vi "nanocal -- nuclear schottky fit -- 2x2 -- V9.vi"() -> ()   [LabVIEW 2021] (continued)
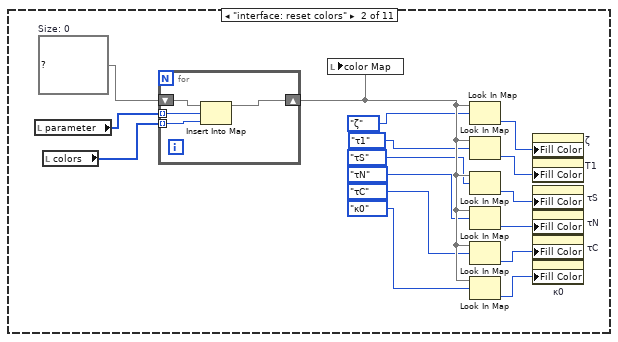
[diagram p3: hidden frame]
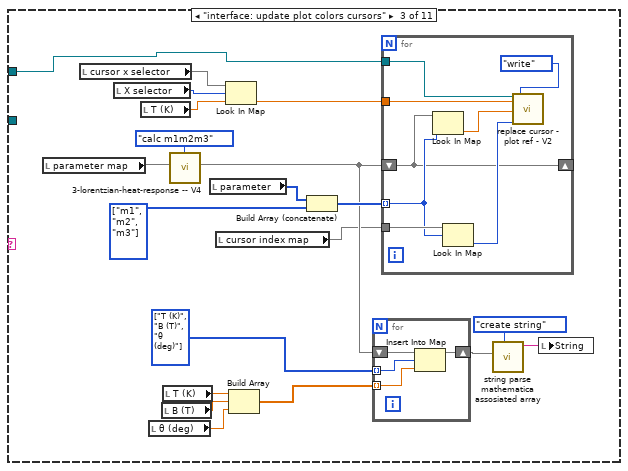
[diagram p4: hidden frame]
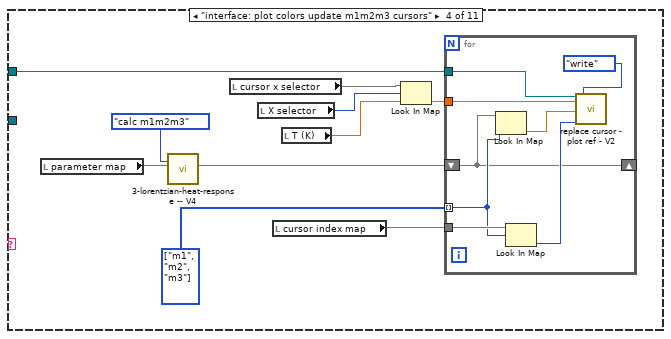
[diagram p5: hidden frame]
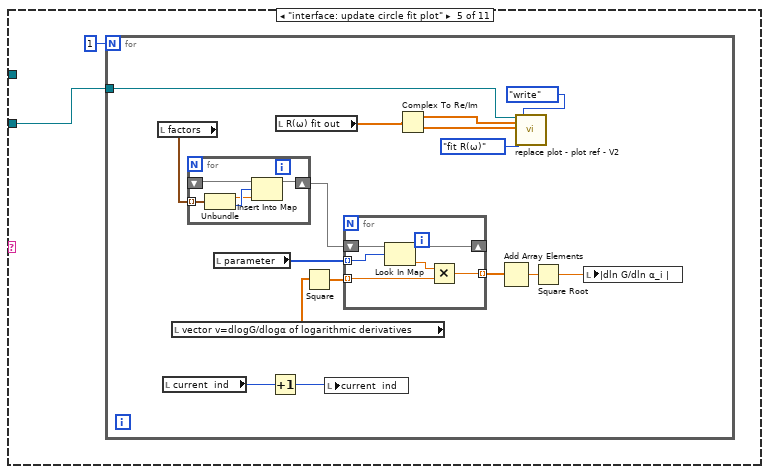
[diagram p6: hidden frame]
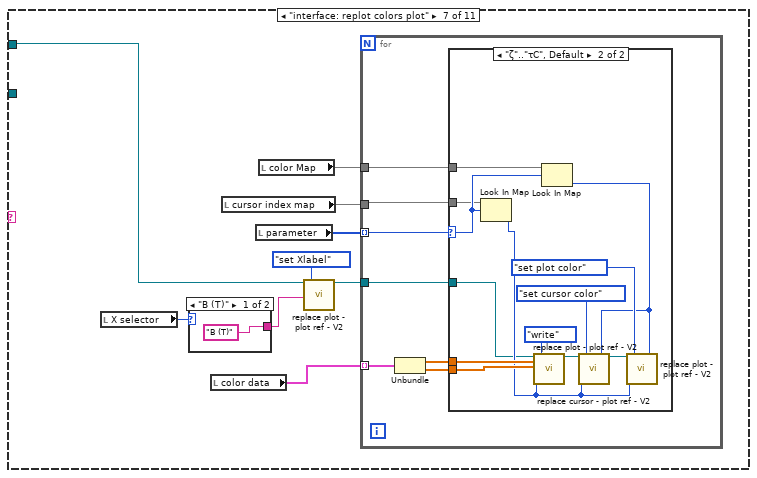
[diagram p8: hidden frame]
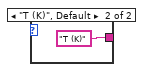
[diagram p9: hidden frame]
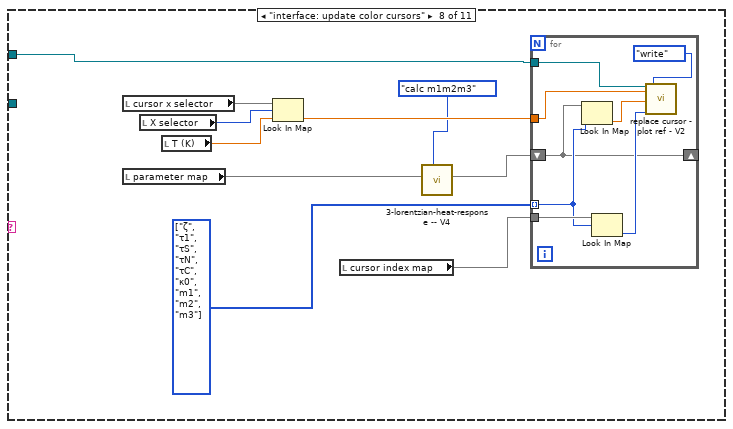
[diagram p11: hidden frame]
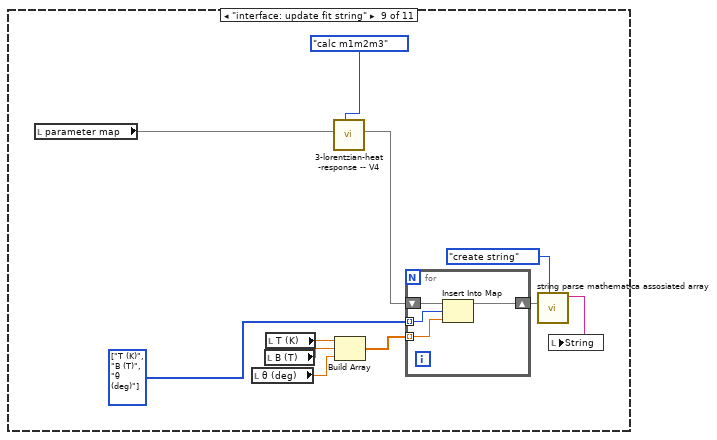
[diagram p12: hidden frame]
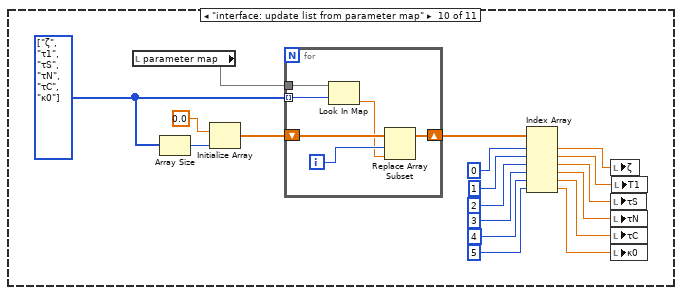
[diagram p13: hidden frame]
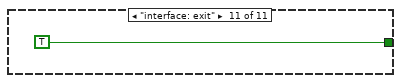
[diagram p14: hidden frame]
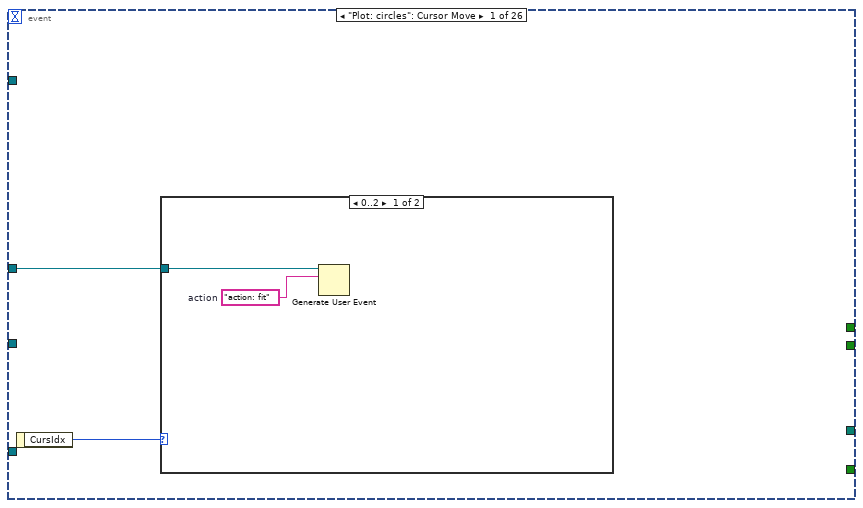
[diagram p15: hidden frame]
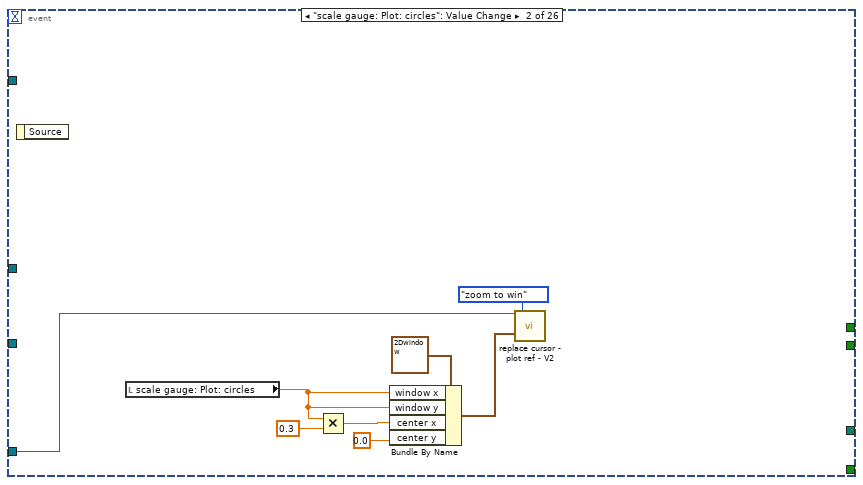
[diagram p17: hidden frame]
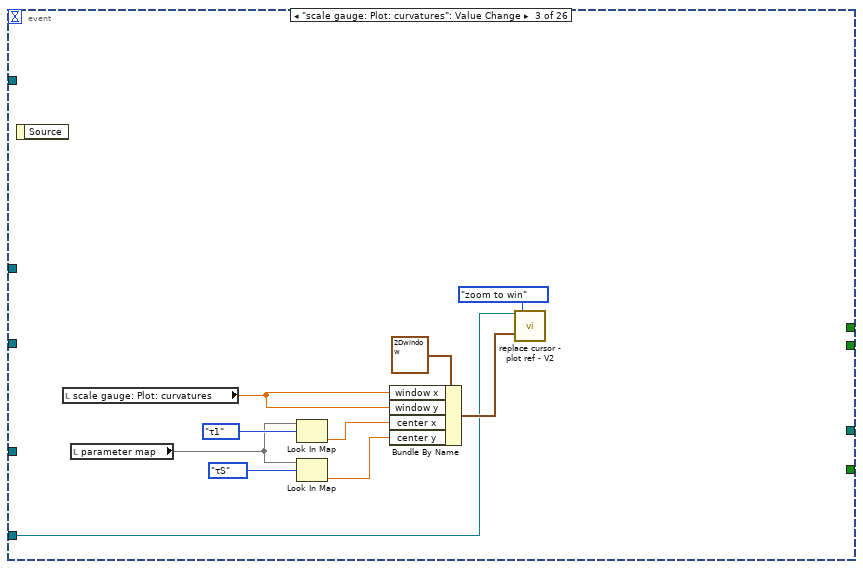
[diagram p18: hidden frame]
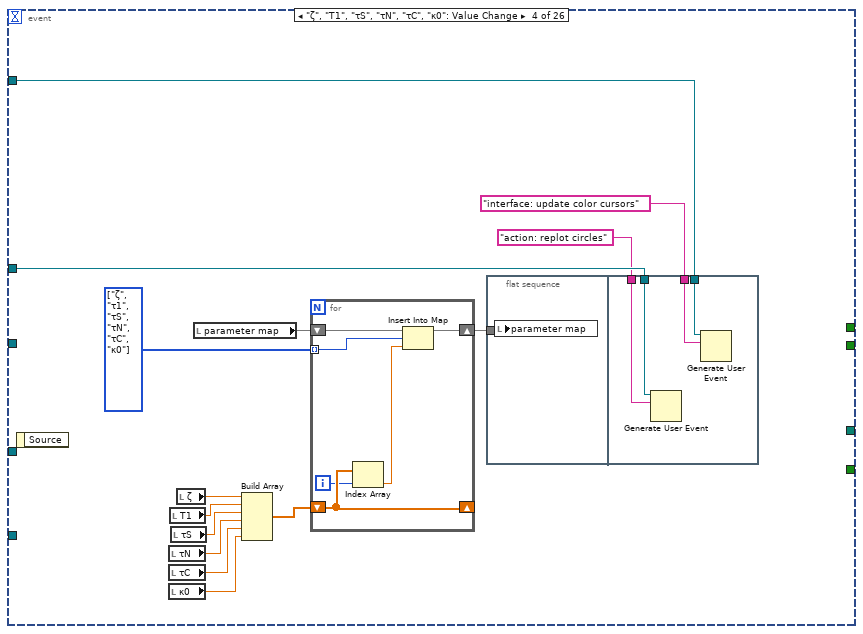
[diagram p19: hidden frame]
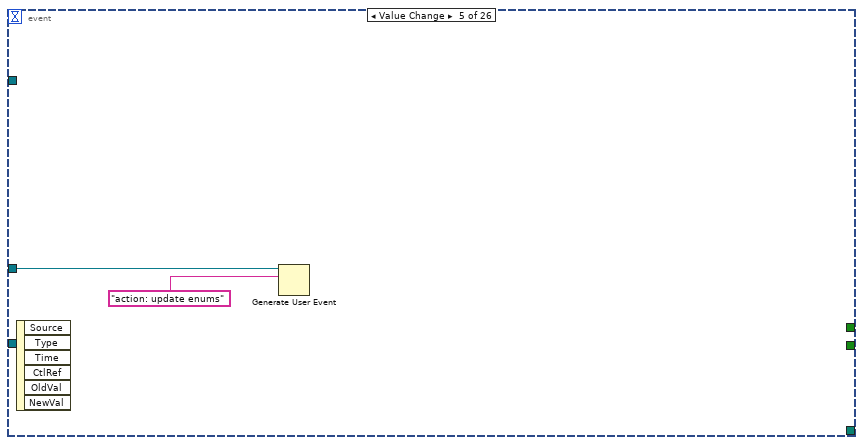
[diagram p20: hidden frame]
            n551 = call "3-lorentzian-heat-response -- V4.vi"("action"=3-lorentzian-heat-response_action."calc m1m2m3", "Map IN"=w1167) -> ("Map OUT"=w1166:map{T2, dbl})  [unwired: 7 in, 2 out]
            n552 = local read "cursor x selector"() -> (w1161:map{T2, dbl})
            n553 = local read "X selector"() -> (w1162:T2)
            n554 = local read "cursor index map"() -> (w1165:map{T2, i32})
            n555 = local read "T (K)"() -> (w1163:dbl)
            n556 = Look In Map(map=w1161, key=w1162, default value=w1163) -> (value=w1164:dbl)  [unwired: 1 out]
            n557 = for {
              tunnel: w1164 -> [w1175]
              tunnel: w1159 -> [w1171] mode=indexing
              tunnel: w1165 -> [w1173]
              shift-right: [w1170] -> _
              shift-left: w1166 -> [w1170]
              tunnel: w1158 -> [w1168]
              n558 = Look In Map(map=w1170, key=w1171) -> (value=w1169:dbl)  [unwired: 1 in, 1 out]
              n559 = Look In Map(map=w1173, key=w1171) -> (value=w1172:i32)  [unwired: 1 in, 1 out]
              n560 = call "replace cursor - plot ref - V2.vi"("Plot ref in"=w1168, "new X"=w1175, "new  Y"=w1169, "cursor index"=w1172, "cursor action"=cursor_action."write") -> ()  [unwired: 11 in, 4 out]
            }
          }
          frame "interface: update circle fit plot" {
            n561 = for {
              N: 1 -> [_]
              tunnel: w1176 -> [w1178]
              n562 = local read "factors"() -> (w1188:cluster{"scaling":dbl, "what":T2}[])
              n563 = local read "current  ind"() -> (w1180:i32)
              n564 = local read "vector v=dlogG/dlogα of logarithmic derivatives"() -> (w1183:dbl[])
              n565 = for {
                shift-right: [w1202] -> w1182
                shift-left: _ -> [w1203]
                tunnel: w1188 -> [w1201] mode=indexing
                n566 = Unbundle(w1201) -> ("scaling"=w1199:dbl, "what"=w1200:T2)
                n567 = Insert Into Map(map in=w1203, key=w1200, value=w1199) -> (map out=w1202:map{T2, dbl})  [unwired: 2 out]
              }
              n568 = local read "parameter"() -> (w1184:T2[])
              n569 = Increment(x=w1180) -> (x+1=w1179:i32)
              n570 = local read "R(ω) fit out"() -> (w1193:cdb[])
              n571 = Square(x=w1183) -> (x^2=w1186:dbl[])
              n572 = local write "current  ind"(w1179) -> ()
              n573 = for {
                tunnel: w1184 -> [w1198] mode=indexing
                shift-right: [w1197] -> _
                shift-left: w1182 -> [w1197]
                tunnel: w1186 -> [w1195] mode=indexing
                tunnel: [w1194] -> w1185 mode=indexing
                n574 = Look In Map(map=w1197, key=w1198) -> (value=w1196:dbl)  [unwired: 1 in, 1 out]
                n575 = Multiply(x=w1196, y=w1195) -> (x*y=w1194:dbl)
              }
              n576 = Complex To Re/Im(x + iy=w1193) -> (x=w1191:dbl[], y=w1192:dbl[])
              n577 = Add Array Elements(numeric array=w1185) -> (sum=w1187:dbl)
              n578 = call "replace plot - plot ref - V2.vi"("Plot ref in"=w1178, "Array X IN"=w1191, "Array Y IN"=w1192, "plot index"=enum16{"data R(ω)", "fit R(ω)"}."fit R(ω)" ("Plost: sweep window"), "cursor action"=cursor_action."write") -> ()  [unwired: 11 in, 4 out]
              n579 = Square Root(x=w1187) -> (sqrt(x)=w1181:dbl)
              n580 = local write "|dln G/dln α_i |"(w1181) -> ()
            }
          }
          frame "interface: update curvature plot" {
            n581 = local read "error goodness weighting"() -> (w1205:T5)
            n582 = local read "newton parameters"() -> (w1206:T3)
            n583 = Bundle By Name(cluster=w1206, "weighting"=w1205) -> (w1204:T3)
            n584 = control-ref of="Plot: curvature"() -> (w1208:refnum<vi>)
            n585 = case shown="True" "update  as you fit" {
              tunnel: w1208 -> [_ _]
              tunnel: w1204 -> [_ w1213]
              frame False {
              }
              frame True {
                n586 = local read "curvature triplets"() -> (w1216:T11[])
                n587 = local read "parameter map"() -> (w1218:map{T2, dbl})
                n588 = local read "sampling size(%)"() -> (w1214:dbl)
                n589 = local read "error-mode"() -> (w1209:T15)
                n590 = call "nanocal -- publish -- freq scan V2.vi"("publisher action"=publisher_action."get") -> ("data"=w1215:T34)  [unwired: 7 in, 3 out]
                n591 = call "nanocal -- generate 3D curvature ellipsoid --  V4.vi"("sampling vicinity size (%)"=w1214, "error mode"=w1209, "newton parameters"=w1213, "data"=w1215, "Curvature triplet array IN"=w1216, "parameter map"=w1218) -> ("Curvature triplet array OUT"=w1212:T11[])  [unwired: 5 in]
                n592 = Index Array(array=w1212, index=0) -> (element=w1210:T11)
                n593 = Unbundle By Name(w1210) -> ()  [unwired: 1 out]
                n594 = local write "curvature triplets"(w1212) -> ()
              }
            }
          }
          frame "interface: replot colors plot" {
            n595 = local read "X selector"() -> (w1220:T2)
            n596 = case shown="\"B (T)\"" w1220 {
              tunnel: ["B (T)" "T (K)"] -> w1226
              frame "B (T)" {
              }
              frame "T (K)", Default {
              }
            }
            n597 = local read "color data"() -> (w1223:cluster{"Array":dbl[], "Array":dbl[]}[])
            n598 = local read "cursor index map"() -> (w1221:map{T2, i32})
            n599 = local read "parameter"() -> (w1227:T2[])
            n600 = local read "color Map"() -> (w1222:map{T2, u32})
            n601 = call "replace plot - plot ref - V2.vi"("Plot ref in"=w1219, "text"=w1226, "cursor action"=cursor_action."set Xlabel") -> ("Plot ref out"=w1224:refnum<vi>)  [unwired: 13 in, 3 out]
            n602 = for {
              tunnel: w1227 -> [w1236] mode=indexing
              tunnel: w1224 -> [w1235]
              tunnel: w1223 -> [w1234] mode=indexing
              tunnel: w1222 -> [w1231]
              tunnel: w1221 -> [w1230]
              n603 = Unbundle(w1234) -> ("Array"=w1232:dbl[], "Array"=w1233:dbl[])
              n604 = case shown="\"ζ\"..\"τC\", Default" w1236 {
                selector: w1236 -> [_ w1245]
                tunnel: w1232 -> [_ w1247]
                tunnel: w1233 -> [_ w1246]
                tunnel: w1231 -> [_ w1244]
                tunnel: w1230 -> [_ w1243]
                tunnel: w1235 -> [_ w1237]
                frame "κ0" {
                }
                frame "ζ".."τC", Default {
                  n605 = Look In Map(map=w1243, key=w1245) -> (value=w1239:i32)  [unwired: 1 in, 1 out]
                  n606 = call "replace plot - plot ref - V2.vi"("Plot ref in"=w1237, "Array X IN"=w1247, "Array Y IN"=w1246, "plot index"=w1239, "cursor action"=cursor_action."write") -> ("Plot ref out"=w1242:refnum<vi>)  [unwired: 11 in, 3 out]
                  n607 = Look In Map(map=w1244, key=w1245) -> (value=w1238:u32)  [unwired: 1 in, 1 out]
                  n608 = call "replace cursor - plot ref - V2.vi"("Plot ref in"=w1242, "cursor index"=w1239, "cursor action"=cursor_action."set cursor color", "Color Box"=w1238) -> ("Plot ref out"=w1241:refnum<vi>)  [unwired: 12 in, 3 out]
                  n609 = call "replace plot - plot ref - V2.vi"("Plot ref in"=w1241, "plot index"=w1239, "cursor action"=cursor_action."set plot color", "Color Box"=w1238) -> ()  [unwired: 12 in, 4 out]
                }
              }
            }
          }
          frame "interface: update color cursors" {
            w1252 = T2[] [enum."ζ", enum."τ1", enum."τS", enum."τN", enum."τC", enum."κ0", enum."m1", enum."m2", enum."m3"] items=["ζ", "τ1", "τS", "τN", "τC", "κ0", "m1", "m2", "m3", "T (K)", "B (T)", "θ (deg)", "side (S|R)", "set of (B|T)", "Re(offset)", "Im(offset)", "στ1", "στ1-", "στ1+", "στS", "στS-", "στS+", "στN", "στN-", "στN+", "τ11", "τ12", "τ21", "τ22", "τN1", "τN2"]
            n610 = local read "cursor x selector"() -> (w1254:map{T2, dbl})
            n611 = local read "parameter map"() -> (w1251:map{T2, dbl})
            n612 = local read "X selector"() -> (w1255:T2)
            n613 = local read "T (K)"() -> (w1256:dbl)
            n614 = Look In Map(map=w1254, key=w1255, default value=w1256) -> (value=w1257:dbl)  [unwired: 1 out]
            n615 = local read "cursor index map"() -> (w1258:map{T2, i32})
            n616 = call "3-lorentzian-heat-response -- V4.vi"("action"=3-lorentzian-heat-response_action."calc m1m2m3", "Map IN"=w1251) -> ("Map OUT"=w1259:map{T2, dbl})  [unwired: 7 in, 2 out]
            n617 = for {
              tunnel: w1257 -> [w1267]
              tunnel: w1250 -> [w1266]
              tunnel: w1252 -> [w1262] mode=indexing
              tunnel: w1258 -> [w1264]
              shift-right: [w1261] -> _
              shift-left: w1259 -> [w1261]
              n618 = Look In Map(map=w1261, key=w1262) -> (value=w1260:dbl)  [unwired: 1 in, 1 out]
              n619 = Look In Map(map=w1264, key=w1262) -> (value=w1263:i32)  [unwired: 1 in, 1 out]
              n620 = call "replace cursor - plot ref - V2.vi"("Plot ref in"=w1266, "new X"=w1267, "new  Y"=w1260, "cursor index"=w1263, "cursor action"=cursor_action."write") -> ()  [unwired: 11 in, 4 out]
            }
          }
          frame "interface: update fit string" {
            w1270 = T2[] [enum."T (K)", enum."B (T)", enum."θ (deg)"] items=["ζ", "τ1", "τS", "τN", "τC", "κ0", "m1", "m2", "m3", "T (K)", "B (T)", "θ (deg)", "side (S|R)", "set of (B|T)", "Re(offset)", "Im(offset)", "στ1", "στ1-", "στ1+", "στS", "στS-", "στS+", "στN", "στN-", "στN+", "τ11", "τ12", "τ21", "τ22", "τN1", "τN2"]
            n621 = local read "parameter map"() -> (w1268:map{T2, dbl})
            n622 = local read "θ (deg)"() -> (w1274:dbl)
            n623 = local read "B (T)"() -> (w1273:dbl)
            n624 = local read "T (K)"() -> (w1272:dbl)
            n625 = call "3-lorentzian-heat-response -- V4.vi"("action"=3-lorentzian-heat-response_action."calc m1m2m3", "Map IN"=w1268) -> ("Map OUT"=w1275:map{T2, dbl})  [unwired: 7 in, 2 out]
            n626 = Build Array(w1272, w1273, w1274) -> (w1276:dbl[])
            n627 = for {
              shift-right: [w1281] -> w1277
              shift-left: w1275 -> [w1282]
              tunnel: w1270 -> [w1280] mode=indexing
              tunnel: w1276 -> [w1279] mode=indexing
              n628 = Insert Into Map(map in=w1282, key=w1280, value=w1279) -> (map out=w1281:map{T2, dbl})  [unwired: 2 out]
            }
            n629 = call "string parse mathematica assosiated array.vi"("action"=mathematica_string_map_action."create string" ("derivative"), "map IN"=w1277) -> ("String OUT"=w1278:string)  [unwired: 8 in, 1 out]
            n630 = local write "String"(w1278) -> ()
          }
          frame "interface: update list from parameter map" {
            w1284 = T2[] [enum."ζ", enum."τ1", enum."τS", enum."τN", enum."τC", enum."κ0"] items=["ζ", "τ1", "τS", "τN", "τC", "κ0", "m1", "m2", "m3", "T (K)", "B (T)", "θ (deg)", "side (S|R)", "set of (B|T)", "Re(offset)", "Im(offset)", "στ1", "στ1-", "στ1+", "στS", "στS-", "στS+", "στN", "στN-", "στN+", "τ11", "τ12", "τ21", "τ22", "τN1", "τN2"]
            n631 = local read "parameter map"() -> (w1287:map{T2, dbl})
            n632 = Array Size(array=w1284) -> (size(s)=w1283:i32)
            n633 = Initialize Array(0.0 ("new X"), w1283) -> (w1286:dbl[])
            n634 = for {
              tunnel: w1284 -> [w1305] mode=indexing
              tunnel: w1287 -> [w1306]
              shift-right: [w1303] -> w1289
              shift-left: w1286 -> [w1304]
              i -> [w1302]
              n635 = Look In Map(map=w1306, key=w1305) -> (value=w1301:dbl)  [unwired: 1 in, 1 out]
              n636 = Replace Array Subset(array=w1304, new element=w1301, index=w1302) -> (w1303:dbl[])
            }
            n637 = Index Array(array=w1289, index #1=0 ("index"), index #2=1 ("index"), index #3=2 ("index"), index #4=3 ("index"), index #5=4 ("index"), index #6=5 ("index")) -> (element #1=w1288:dbl, element #2=w1296:dbl, element #3=w1297:dbl, element #4=w1298:dbl, element #5=w1299:dbl, element #6=w1300:dbl)
            n638 = local write "ζ"(w1288) -> ()
            n639 = local write "τS"(w1297) -> ()
            n640 = local write "τN"(w1298) -> ()
            n641 = local write "τC"(w1299) -> ()
            n642 = local write "κ0"(w1300) -> ()
            n643 = local write "T1"(w1296) -> ()
          }
          frame "interface: exit" {
          }
        }
      }
    }
  }
  n644 = while "interface events" {
    tunnel: w9 -> [w1313]
    tunnel: w38 -> [w1312]
    tunnel: w35 -> [w1311]
    tunnel: w10 -> [w1310]
    tunnel: w3 -> [w1308]
    stop <- FALSE stop-if-true
    n645 = event shown="[11] \"offset Re offset Im\", \"|ω| < limit (Hz)\", \"cspan\": Value Change" {
      selector: _ -> [_ _ _ _ _ _ _ _ _ _ _ _ _ _ _ _ _ _ _ _ _ _ _ _ _ _]
      dyn-events: _ -> [_ _ _ _ _ _ _ _ _ _ _ _ _ _ _ _ _ _ _ _ _ _ _ _ _ _]
      timeout: _ -> [_ _ _ _ _ _ _ _ _ _ _ _ _ _ _ _ _ _ _ _ _ _ _ _ _ _]
      tunnel: w1313 -> [w1314 _ _ w1337 w1361 _ w1386 w1392 _ w1396 w1398 w1400 w1403 w1410 w1506 w1527 w1547 w1549 w1553 w1556 w1559 w1562 w1570 w1574 w1576 w1579]
      tunnel: [_ _ _ _ _ _ _ _ _ "load! :l" _ _ _ _ _ _ _ _ _ _ _ _ _ _ _ _] -> _
      tunnel: [_ _ _ _ _ _ "go / pause!" _ _ _ _ _ "parse! :p" _ _ _ "Math→τ! :q" _ "τ→Math! :p" "Math→ string OUT! :s" "generate empty string from filelist !" "string IN → Math!" _ _ "plot landscape!" _] -> _
      tunnel: w1312 -> [_ w1318 _ _ _ w1363 _ _ _ _ _ _ _ w1406 _ _ _ _ _ _ _ _ _ _ _ _]
      tunnel: w1311 -> [_ _ _ _ _ _ _ _ _ _ _ _ _ _ w1514 w1535 _ _ _ _ _ _ _ _ _ _]
      tunnel: [_ _ _ _ _ _ _ _ _ _ "Read from file" _ _ _ _ _ _ _ _ _ _ _ _ _ _ _] -> _
      tunnel: [_ _ _ _ _ _ _ _ _ _ _ _ _ _ _ _ _ "load default values" _ _ _ _ _ _ _ _] -> _
      tunnel: w1310 -> [_ _ _ w1339 _ _ _ _ _ _ _ _ _ _ w1504 w1525 _ _ _ _ _ _ _ _ _ _]
      tunnel: w1308 -> [_ _ w1332 _ _ _ _ _ _ _ _ _ _ w1405 _ _ _ _ _ _ _ _ _ _ _ _]
      event "Plot: circles": Cursor Move {
        n646 = event-data() -> ("CursIdx"=w1315:i32)  [unwired: 1 in]
        n647 = case shown="0..2" w1315 {
          tunnel: w1314 -> [w1317 _]
          frame 0..2 {
            w1316 = "action: fit"  # action
            n648 = Generate User Event(user event=w1317, event data cluster=w1316) -> ()  [unwired: 2 in, 2 out]
          }
          frame 3..5, Default {
          }
        }
      }
      event "scale gauge: Plot: circles": Value Change {
        n649 = event-data() -> ()  [unwired: 1 in, 1 out]
        n650 = local read "scale gauge: Plot: circles"() -> (w1324:dbl)
        n651 = Multiply(x=w1324, y=0.3) -> (x*y=w1325:dbl)
        n652 = Bundle By Name(cluster=T37 {"window y"=0.0021014740628288917, "center x"=44850.89441339177, "center y"=2.5658109925320947, "window x"=17480.201988350764} ("window IN"), "window x"=w1324, "window y"=w1324, "center x"=w1325, "center y"=0.0) -> (w1323:T37)
        n653 = call "replace cursor - plot ref - V2.vi"("Plot ref in"=w1318, "window IN"=w1323, "cursor action"=cursor_action."zoom to win") -> ()  [unwired: 13 in, 4 out]
      }
      event "scale gauge: Plot: curvatures": Value Change {
        n654 = event-data() -> ()  [unwired: 1 in, 1 out]
        n655 = local read "scale gauge: Plot: curvatures"() -> (w1328:dbl)
        n656 = local read "parameter map"() -> (w1329:map{T2, dbl})
        n657 = Look In Map(map=w1329, key=3-lorentzian-parameters."τ1") -> (value=w1327:dbl)  [unwired: 1 in, 1 out]
        n658 = Look In Map(map=w1329, key=3-lorentzian-parameters."τS") -> (value=w1326:dbl)  [unwired: 1 in, 1 out]
        n659 = Bundle By Name(cluster=T37 {"window y"=0.0021014740628288917, "center x"=44850.89441339177, "center y"=2.5658109925320947, "window x"=17480.201988350764} ("window IN"), "window x"=w1328, "window y"=w1328, "center x"=w1327, "center y"=w1326) -> (w1335:T37)
        n660 = call "replace cursor - plot ref - V2.vi"("Plot ref in"=w1332, "window IN"=w1335, "cursor action"=cursor_action."zoom to win") -> ()  [unwired: 13 in, 4 out]
      }
      event "ζ", "T1", "τS", "τN", "τC", "κ0": Value Change {
        w1340 = T2[] [enum."ζ", enum."τ1", enum."τS", enum."τN", enum."τC", enum."κ0"] items=["ζ", "τ1", "τS", "τN", "τC", "κ0", "m1", "m2", "m3", "T (K)", "B (T)", "θ (deg)", "side (S|R)", "set of (B|T)", "Re(offset)", "Im(offset)", "στ1", "στ1-", "στ1+", "στS", "στS-", "στS+", "στN", "στN-", "στN+", "τ11", "τ12", "τ21", "τ22", "τN1", "τN2"]
        n661 = event-data() -> ()  [unwired: 1 in, 1 out]
        n662 = local read "τN"() -> (w1346:dbl)
        n663 = local read "τC"() -> (w1345:dbl)
        n664 = local read "κ0"() -> (w1344:dbl)
        n665 = local read "T1"() -> (w1348:dbl)
        n666 = local read "τS"() -> (w1347:dbl)
        n667 = local read "ζ"() -> (w1349:dbl)
        n668 = local read "parameter map"() -> (w1341:map{T2, dbl})
        n669 = Build Array(w1349, w1348, w1347, w1346, w1345, w1344) -> (w1343:dbl[])
        n670 = for {
          tunnel: w1340 -> [w1355] mode=indexing
          shift-right: [w1360] -> _
          shift-left: w1343 -> [w1360]
          shift-right: [w1357] -> w1342
          shift-left: w1341 -> [w1358]
          i -> [w1359]
          n671 = Index Array(array=w1360, index=w1359) -> (element=w1356:dbl)
          n672 = Insert Into Map(map in=w1358, key=w1355, value=w1356) -> (map out=w1357:map{T2, dbl})  [unwired: 2 out]
        }
        n673 = flat-sequence {
          tunnel: w1342 -> [w1350]
          tunnel: w1339 -> [w1354]
          tunnel: "interface: update color cursors" ("event data") -> [w1353]
          tunnel: w1337 -> [w1352]
          tunnel: "action: replot circles" ("event data") -> [w1351]
          frame #0 {
            n674 = local write "parameter map"(w1350) -> ()
          }
          frame #1 {
            n675 = Generate User Event(user event=w1352, event data cluster=w1351) -> ()  [unwired: 2 in, 2 out]
            n676 = Generate User Event(user event=w1354, event data cluster=w1353) -> ()  [unwired: 2 in, 2 out]
          }
        }
      }
      event Value Change {
        n677 = event-data() -> ()  [unwired: 1 in, 6 out]
        n678 = Generate User Event(user event=w1361, event data cluster="action: update enums" ("event data")) -> ()  [unwired: 2 in, 2 out]
      }
      event "ω0 (rad/sec)": Value Change {
        n679 = event-data() -> ()  [unwired: 1 in, 1 out]
        n680 = local read "parameter map"() -> (w1365:map{T2, dbl})
        n681 = call "nanocal -- publish -- freq scan V2.vi"("publisher action"=publisher_action."get") -> ("z out (V)"=w1383:cdb[], "ω out (Hz)"=w1378:dbl[])  [unwired: 7 in, 2 out]
        n682 = Divide(x="ω0 (rad/sec)", y=6.283185307179586) -> (x/y=w1376:dbl)
        n683 = call "3-lorentzian-heat-response -- V4.vi"("action"=3-lorentzian-heat-response_action."calc R", "Map IN"=w1365, "omega IN (rad/sec)"="ω0 (rad/sec)") -> ("Romega"=w1375:cdb)  [unwired: 6 in, 2 out]
        n684 = Threshold 1D Array(2:w1376, 3:w1378) -> (0:w1377:dbl)  [unwired: 1 in]
        n685 = Complex To Re/Im(x + iy=w1375) -> (x=w1373:dbl, y=w1374:dbl)
        n686 = Index Array(array=w1383, index=w1377) -> (element=w1380:cdb)
        n687 = call "replace cursor - plot ref - V2.vi"("Plot ref in"=w1363, "new X"=w1373, "new  Y"=w1374, "cursor index"=0, "cursor action"=cursor_action."write") -> ("Plot ref out"=w1379:refnum<vi>)  [unwired: 11 in, 3 out]
        n688 = Complex To Re/Im(x + iy=w1380) -> (x=w1381:dbl, y=w1382:dbl)
        n689 = call "replace cursor - plot ref - V2.vi"("Plot ref in"=w1379, "new X"=w1381, "new  Y"=w1382, "cursor index"=1, "cursor action"=cursor_action."write") -> ()  [unwired: 11 in, 4 out]
      }
      event "go / pause!": Value Change {
        n690 = event-data() -> ()  [unwired: 1 in, 1 out]
        n691 = local read "newton is active"() -> (w1384:bool)
        n692 = case shown="True" w1384 {
          tunnel: w1386 -> [_ w1391]
          tunnel: [FALSE TRUE] -> w1385
          frame True {
          }
          frame False {
            n693 = Generate User Event(user event=w1391, event data cluster="action: gradient step" ("event data")) -> ()  [unwired: 2 in, 2 out]
          }
        }
        n694 = local write "newton is active"(w1385) -> ()
      }
      event "selector": Value Change {
        n695 = event-data() -> ()  [unwired: 1 in, 1 out]
        n696 = Generate User Event(user event=w1392, event data cluster="action: update state of selectors" ("event data")) -> ()  [unwired: 2 in, 2 out]
      }
      event "Plot: circles": Cursor Release {
        n697 = event-data() -> ()  [unwired: 1 in, 1 out]
      }
      event "load! :l": Value Change {
        n698 = event-data() -> ()  [unwired: 1 in, 6 out]
        n699 = Generate User Event "action User Event"(user event=w1396, event data cluster="action: read from file" ("event data")) -> ()  [unwired: 2 in, 2 out]
      }
      event "Read from file": Value Change {
        n700 = event-data() -> ()  [unwired: 1 in, 6 out]
        n701 = Generate User Event ("action User Event")(user event=w1398, event data cluster="action: read from file" ("event data")) -> ()  [unwired: 2 in, 2 out]
      }
      event "offset Re\noffset Im", "|ω| < limit (Hz)", "cspan": Value Change {
        n702 = event-data() -> ()  [unwired: 1 in, 6 out]
        n703 = Generate User Event "action User Event"(user event=w1400, event data cluster="action: read from file" ("event data")) -> ()  [unwired: 2 in, 2 out]
      }
      event "parse! :p": Value Change {
        n704 = event-data() -> ()  [unwired: 1 in, 6 out]
        n705 = Generate User Event "action User Event"(user event=w1403, event data cluster="action: parse string" ("event data")) -> ()  [unwired: 2 in, 2 out]
      }
      event Key Down {
        n706 = event-data() -> ("Char"=w1408:i16, "VKey"=w1411:T38)  [unwired: 1 in]
        n707 = Build Array(w1408) -> (w1409:i16[])
        n708 = Byte Array To String(unsigned byte array=w1409) -> (string=w1407:string)
        n709 = case shown="\"ASCII\", Default" w1411 {
          selector: w1411 -> [_ _ _ _ _ w1498]
          tunnel: w1410 -> [w1415 _ w1491 _ _ _]
          tunnel: w1407 -> [w1414 _ _ _ _ _]
          tunnel: w1406 -> [w1413 _ _ _ _ w1497]
          tunnel: w1405 -> [w1412 _ _ _ _ w1496]
          frame "ASCII", Default {
            n710 = case shown="\"b\"" w1414 {
              selector: w1414 -> [_ _ _ _ _ _ w1440 w1450 _ _ _ _ w1470 _]
              tunnel: w1415 -> [_ _ w1416 w1418 w1422 _ _ _ _ w1461 w1464 w1466 w1468 w1489]
              tunnel: w1413 -> [_ _ _ _ _ w1436 _ _ _ _ _ _ _ _]
              tunnel: w1412 -> [_ _ _ _ _ w1429 _ _ _ _ _ _ _ _]
              frame "0", Default {
              }
              frame "a" {
              }
              frame "s" {
                n711 = Generate User Event(user event=w1416, event data cluster="action: write mathematica string" ("event data")) -> ()  [unwired: 2 in, 2 out]
              }
              frame "l" {
                n712 = Generate User Event(user event=w1418, event data cluster="action: read from file" ("event data")) -> ()  [unwired: 2 in, 2 out]
              }
              frame " " {
                n713 = local read "newton is active"() -> (w1421:bool)
                n714 = case shown="False" w1421 {
                  selector: w1421 -> [w1424 w1426]
                  tunnel: w1422 -> [_ w1428]
                  tunnel: [w1423 w1425] -> w1420
                  frame True {
                    n715 = Not(x=w1424) -> (.not. x?=w1423:bool)
                  }
                  frame False {
                    n716 = Generate User Event(user event=w1428, event data cluster="action: gradient step" ("event data")) -> ()  [unwired: 2 in, 2 out]
                    n717 = Not(x=w1426) -> (.not. x?=w1425:bool)
                  }
                }
                n718 = local write "newton is active"(w1420) -> ()
              }
              frame "?" {
                # "?"
                n719 = call "replace cursor - plot ref - V2.vi"("Plot ref in"=w1436, "cursor action"=cursor_action."zoom to win") -> ("Plot ref out"=w1435:refnum<vi>)  [unwired: 14 in, 3 out]
                n720 = call "replace cursor - plot ref - V2.vi"("Plot ref in"=w1435, "cursor action"=cursor_action."smart zoom out&aspect") -> ()  [unwired: 14 in, 4 out]
                n721 = call "replace cursor - plot ref - V2.vi"("Plot ref in"=w1429, "cursor action"=cursor_action."zoom to win") -> ("Plot ref out"=w1432:refnum<vi>)  [unwired: 14 in, 3 out]
                n722 = call "replace cursor - plot ref - V2.vi"("Plot ref in"=w1432, "cursor action"=cursor_action."smart zoom out&aspect") -> ()  [unwired: 14 in, 4 out]
              }
              frame ",", "." {
                n723 = local read "newton parameters"() -> (w1438:T3)
                n724 = case shown="\".\"" w1440 {
                  tunnel: [0.7 1.0 1.5] -> w1439
                  frame "," {
                  }
                  frame "0", Default {
                  }
                  frame "." {
                  }
                }
                n725 = in-place {
                  in-place-border: w1439 -> [w1443]
                  n726 = in-place-cluster #7(w1438) -> ("PID-P"=w1441:dbl)
                  n727 = Multiply(x=w1443, y=w1441) -> (x*y=w1442:dbl)
                  n728 = in-place-cluster #7("PID-P"=w1442) -> (w1437:T3)
                }
                n729 = local write "newton parameters"(w1437) -> ()
              }
              frame "<", ">" {
                n730 = local read "newton parameters"() -> (w1448:T3)
                n731 = case shown="\"<\"" w1450 {
                  tunnel: [-5 0 5] -> w1449
                  frame "<" {
                  }
                  frame "0", Default {
                  }
                  frame ">" {
                  }
                }
                n732 = in-place {
                  in-place-border: w1449 -> [w1456]
                  n733 = in-place-cluster #8(w1448) -> ("PID-I"=w1455:i32)
                  n734 = Add(x=w1456, y=w1455) -> (x+y=w1454:i32)
                  n735 = In Range and Coerce(upper limit=100, x=w1454, lower limit=2) -> (coerced(x)=w1451:i32)  [unwired: 1 out]
                  n736 = in-place-cluster #8("PID-I"=w1451) -> (w1447:T3)
                }
                n737 = local write "newton parameters"(w1447) -> ()
              }
              frame "b" {
                n738 = local read "String"() -> (w1460:string)
                n739 = local write "backup string :b"(w1460) -> ()
              }
              frame "u" {
                n740 = Generate User Event(user event=w1461, event data cluster="ignoreaction: uco" ("event data")) -> ()  [unwired: 2 in, 2 out]
              }
              frame "p" {
                n741 = Generate User Event ("action User Event")(user event=w1464, event data cluster="action: copy to math" ("event data")) -> ()  [unwired: 2 in, 2 out]
              }
              frame "q" {
                n742 = Generate User Event ("action User Event")(user event=w1466, event data cluster="action: copy from math" ("event data")) -> ()  [unwired: 2 in, 2 out]
              }
              frame "\\", "|" {
                n743 = for {
                  N: 1 -> [_]
                  tunnel: w1470 -> [w1484]
                  tunnel: w1468 -> [w1483]
                  tunnel: [w1483] -> w1467
                  n744 = local read "selection :|\\"() -> (w1476:u16)
                  n745 = property on="selection :|\\" class="Ring (strict)"() -> ("NumItems"=w1474:u32)  [unwired: 2 in, 2 out]
                  n746 = To Long Integer(number=w1476) -> (32bit integer=w1475:i32)
                  n747 = case shown="\"|\", Default" w1484 {
                    tunnel: w1475 -> [w1486 w1488]
                    tunnel: [w1485 w1487] -> w1480
                    frame "|", Default {
                      n748 = Decrement(x=w1486) -> (x-1=w1485:i32)
                    }
                    frame "\\" {
                      n749 = Increment(x=w1488) -> (x+1=w1487:i32)
                    }
                  }
                  n750 = To Long Integer(number=w1474) -> (32bit integer=w1473:i32)
                  n751 = Greater Or Equal?(x=w1480, y=w1473) -> (x >= y?=w1482:bool)
                  n752 = Select(t=u16 0 ("lower limit"), s=w1482, f=w1480) -> (s? t:f=w1477:i32)
                  n753 = Decrement(x=w1473) -> (x-1=w1478:i32)
                  n754 = Less Than 0?(x=w1477) -> (x < 0?=w1479:bool)
                  n755 = Select(t=w1478, s=w1479, f=w1477) -> (s? t:f=w1472:i32)
                  n756 = local write "selection :|\\"(w1472) -> ()
                }
                n757 = Generate User Event ("action User Event")(user event=w1467, event data cluster="action: constrained filenames select" ("event data")) -> ()  [unwired: 2 in, 2 out]
              }
              frame "m" {
                n758 = Generate User Event ("action User Event")(user event=w1489, event data cluster="action: copy from math" ("event data")) -> ()  [unwired: 2 in, 2 out]
              }
            }
          }
          frame "PageUp" {
          }
          frame "Enter" {
            n759 = Generate User Event ("action User Event")(user event=w1491, event data cluster="action: new sweep" ("event data")) -> (user event out=w1492:refnum<user-event>)  [unwired: 2 in, 1 out]
            n760 = Generate User Event ("action User Event")(user event=w1492, event data cluster="action: replot colors" ("event data")) -> ()  [unwired: 2 in, 2 out]
          }
          frame "Caps" {
          }
          frame "PageDown" {
          }
          frame "Up".."Right" {
            n761 = case shown="\"Down\"" w1498 {
              tunnel: [cursor_action."zoom in 20%" ("cursor action") cursor_action."zoom out 20%" ("cursor action") cursor_action."zoom out 20%" ("cursor action") cursor_action."zoom in 20%" ("cursor action")] -> w1495
              frame "Up", Default {
              }
              frame "Down" {
              }
              frame "Left" {
              }
              frame "Right" {
              }
            }
            n762 = call "replace cursor - plot ref - V2.vi"("Plot ref in"=w1497, "cursor action"=w1495) -> ()  [unwired: 14 in, 4 out]
            n763 = call "replace cursor - plot ref - V2.vi"("Plot ref in"=w1496, "cursor action"=w1495) -> ()  [unwired: 14 in, 4 out]
          }
        }
      }
      event "Plot:  colors": Cursor Move {
        (unwired) "interface: plot colors update m1m2m3 cursors" ("event data")
        n764 = event-data() -> ("CursIdx"=w1512:i32)  [unwired: 1 in]
        n765 = local read "reverse cursor index map"() -> (w1513:map{i32, T2})
        n766 = call "replace cursor - plot ref - V2.vi"("Plot ref in"=w1514, "cursor index"=w1512, "cursor action"=cursor_action."read") -> ("read Y"=w1511:dbl)  [unwired: 13 in, 3 out]
        n767 = local read "parameter map"() -> (w1510:map{T2, dbl})
        n768 = Look In Map(map=w1513, key=w1512) -> (value=w1508:T2)  [unwired: 1 in, 1 out]
        n769 = in-place {
          in-place-border: w1511 -> [w1522]
          in-place-border: LVMapReplaceAction."Modify Entry only if found" ("action") -> [w1521]
          n770 = in-place-map #9(w1510, w1508) -> ()  [unwired: 1 in, 2 out]
          n771 = in-place-map #9(w1522, w1521) -> (w1509:map{T2, dbl})  [unwired: 2 out]
        }
        n772 = flat-sequence {
          tunnel: w1509 -> [w1516]
          tunnel: w1506 -> [w1520]
          tunnel: "action: replot circles" ("event data") -> [w1519]
          tunnel: w1504 -> [w1518]
          tunnel: "interface: update list from parameter map" ("event data") -> [w1517]
          frame #0 {
            n773 = local write "parameter map"(w1516) -> ()
          }
          frame #1 {
            n774 = Generate User Event(user event=w1520, event data cluster=w1519) -> ()  [unwired: 2 in, 2 out]
            n775 = Generate User Event(user event=w1518, event data cluster=w1517) -> ()  [unwired: 2 in, 2 out]
          }
        }
      }
      event "Plot:  colors": Cursor Release {
        n776 = event-data() -> ("CursIdx"=w1533:i32)  [unwired: 1 in]
        n777 = local read "reverse cursor index map"() -> (w1534:map{i32, T2})
        n778 = call "replace cursor - plot ref - V2.vi"("Plot ref in"=w1535, "cursor index"=w1533, "cursor action"=cursor_action."read") -> ("read Y"=w1532:dbl)  [unwired: 13 in, 3 out]
        n779 = local read "parameter map"() -> (w1531:map{T2, dbl})
        n780 = Look In Map(map=w1534, key=w1533) -> (value=w1529:T2)  [unwired: 1 in, 1 out]
        n781 = in-place {
          in-place-border: w1532 -> [w1545]
          in-place-border: LVMapReplaceAction."Modify Entry only if found" ("action") -> [w1544]
          n782 = in-place-map #10(w1531, w1529) -> ()  [unwired: 1 in, 2 out]
          n783 = in-place-map #10(w1545, w1544) -> (w1530:map{T2, dbl})  [unwired: 2 out]
        }
        n784 = flat-sequence {
          tunnel: w1530 -> [w1537]
          tunnel: w1527 -> [w1543]
          tunnel: "action: replot circles" ("event data") -> [w1542]
          tunnel: w1525 -> [w1541]
          tunnel: "interface: update list from parameter map" ("event data") -> [w1540]
          tunnel: "interface: plot colors update m1m2m3 cursors" ("event data") -> [w1538]
          frame #0 {
            n785 = local write "parameter map"(w1537) -> ()
          }
          frame #1 {
            n786 = Generate User Event(user event=w1543, event data cluster=w1542) -> ()  [unwired: 2 in, 2 out]
            n787 = Generate User Event(user event=w1541, event data cluster=w1540) -> (user event out=w1539:refnum<user-event>)  [unwired: 2 in, 1 out]
            n788 = Generate User Event(user event=w1539, event data cluster=w1538) -> ()  [unwired: 2 in, 2 out]
          }
        }
      }
      event "Math→τ! :q": Value Change {
        n789 = event-data() -> ()  [unwired: 1 in, 1 out]
        n790 = Generate User Event(user event=w1547, event data cluster="action: copy from math" ("event data")) -> ()  [unwired: 2 in, 2 out]
      }
      event "load default values": Value Change {
        n791 = event-data() -> ()  [unwired: 1 in, 1 out]
        n792 = Generate User Event(user event=w1549, event data cluster="action: update default values" ("event data")) -> ()  [unwired: 2 in, 2 out]
      }
      event "τ→Math! :p": Value Change {
        n793 = event-data() -> ()  [unwired: 1 in, 1 out]
        n794 = Generate User Event(user event=w1553, event data cluster="action: copy to math" ("event data")) -> ()  [unwired: 2 in, 2 out]
      }
      event "Math→ string OUT! :s": Value Change {
        n795 = event-data() -> ()  [unwired: 1 in, 1 out]
        n796 = Generate User Event(user event=w1556, event data cluster="action: write mathematica string" ("event data")) -> ()  [unwired: 2 in, 2 out]
      }
      event "generate empty string from filelist !": Value Change {
        n797 = event-data() -> ()  [unwired: 1 in, 1 out]
        n798 = Generate User Event(user event=w1559, event data cluster="action: empty string from filelist" ("event data")) -> ()  [unwired: 2 in, 2 out]
      }
      event "string IN → Math!": Value Change {
        n799 = event-data() -> ()  [unwired: 1 in, 1 out]
        n800 = Generate User Event(user event=w1562, event data cluster="action: read mathematica string" ("event data")) -> ()  [unwired: 2 in, 2 out]
      }
      event "filenames": Value Change {
        n801 = event-data() -> ()  [unwired: 1 in, 1 out]
        n802 = local read "filesnames lookup"() -> (w1569:map{i32, string})
        n803 = local read "all full filenames"() -> (w1567:map{string, path})
        n804 = local read "filenames"() -> (w1568:u16)
        n805 = Look In Map(map=w1569, key=w1568) -> (value=w1566:string)  [unwired: 1 in, 1 out]
        n806 = Look In Map(map=w1567, key=w1566) -> (value=w1564:path)  [unwired: 1 in, 1 out]
        n807 = for {
          N: 1 -> [_]
          tunnel: w1570 -> [w1572]
          tunnel: w1564 -> [w1571]
          n808 = local write "Read from file"(w1571) -> ()
          n809 = Generate User Event(user event=w1572, event data cluster="action: read from file" ("event data")) -> ()  [unwired: 2 in, 2 out]
        }
      }
      event "selection :|\\": Value Change {
        n810 = event-data() -> ()  [unwired: 1 in, 1 out]
        n811 = Generate User Event(user event=w1574, event data cluster="action: constrained filenames select" ("event data")) -> ()  [unwired: 2 in, 2 out]
      }
      event "plot landscape!", "range one", "range two": Value Change {
        n812 = event-data() -> ()  [unwired: 1 in, 6 out]
        n813 = Generate User Event(user event=w1576, event data cluster="action: plot landscape" ("event data")) -> ()  [unwired: 2 in, 2 out]
      }
      event "colors": Value Change {
        n814 = event-data() -> ()  [unwired: 1 in, 6 out]
        n815 = Generate User Event(user event=w1579, event data cluster="action: reset colors" ("event data")) -> ()  [unwired: 2 in, 2 out]
      }
    }
  }
  "cursor x selector" <- w36
